vi "Keithley 648X Series Acquire and Enable Relative Values.vi"() -> ()   [LabVIEW 2024]
doc: "This example shows how to configure a measurement and take a reading."
uses:
  <instrlib>/Keithley 648X Series/Keithley 648X Series.lvlib
panel:
  in  "Digital Filter Noise Tolerance":dbl
  in  "Enable Digital Filter":u16(ring) items=["Disable", "Enable", "Advanced"]
  in  "Digital Filter Type":u16(ring) items=["Repeating", "Moving"]
  in  "Digital Filter Count":i32=10
  in  "Median Filter Rank":u16(ring)=1 items=["1"=1, "2"=2, "3"=3, "4"=4, "5"=5]
  in  "Enable Median Filter":bool
  in  "Measurement Time":dbl=6.0
  in  "Trigger Delay":dbl
  in  "Trigger Loop Count":i32=1
  in  "Trigger Source":u16(ring) items=["Immediate", "Tlink"]
  in  "Arm Timer Interval":dbl=0.1
  in  "Arm Loop Count":i32=1
  in  "Arm Source":u16(ring) items=["Immediate", "Timer", "Bus", "Tlink", "Manual", "Negative SOT", "Positive SOT", "Bidirectional SOT"]
  out "Relative Measurements":cluster{dbl[], dbl[]}(graph)
  in  "Serial Configuration":T1={"Baud Rate"=9600, "Parity"=0, "Data Bits"=8, "Stop Bits"=10, "Flow Control"=0} {"Flow Control" items=["None", "XON/XOFF", "RTS/CTS", "XON/XOFF & RTS/CTS", "DTR/DSR", "XON/XOFF & DTR/DSR"]; "Stop Bits" items=["1.0"=10, "1.5"=15, "2.0"=20]; "Data Bits" items=["7"=7, "8"=8]; "Parity" items=["None", "Odd", "Even", "Mark", "Space"]; "Baud Rate" items=["300"=300, "600"=600, "1200"=1200, "2400"=2400, "4800"=4800, "9600"=9600, "19200"=19200]}
  in  "VISA resource name":refnum<visa-resource-name>
  # "(c) 2017 National Instruments.  ALL RIGHTS RESERVED."
  # "Note: The product of Arm Loop Count and Trigger Loop Count cannot exceed the maximum non-infinite value that either control can take."
  # "Configure Data Acquisition"
  # "Configure Data Filtration"
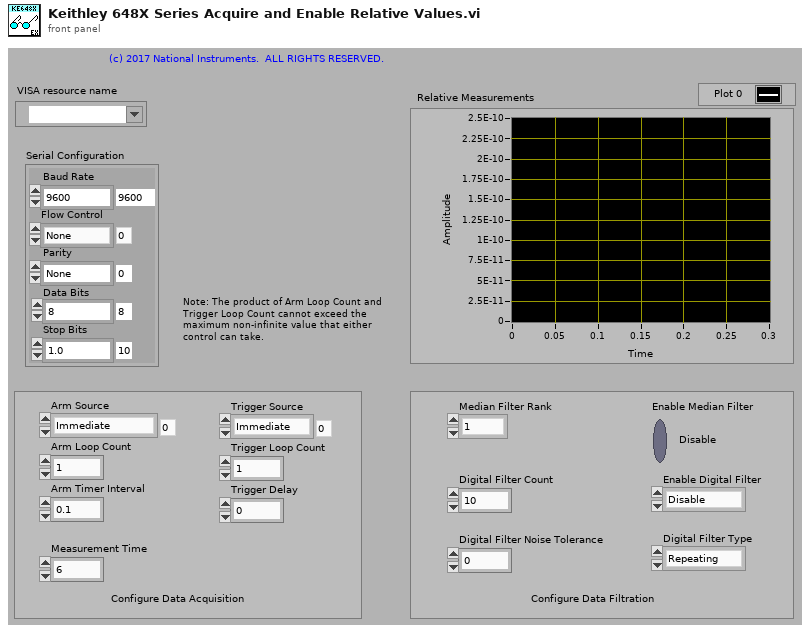
[diagram p1: front panel]
types:
  T1 = cluster{"Baud Rate":u32, "Parity":u16, "Data Bits":u16, "Stop Bits":u16, "Flow Control":u16}
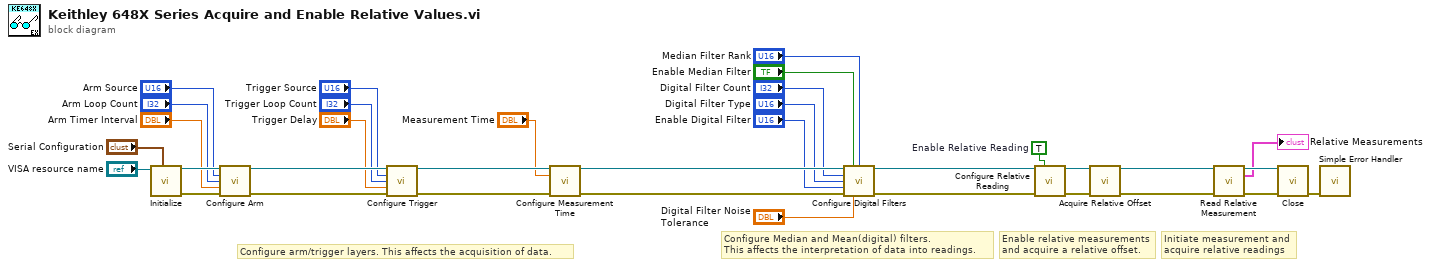
[diagram p0: block diagram]
diagram:
  w20 = TRUE  # Enable Relative Reading
  # "Initiate measurement and\nacquire relative readings"
  # "Enable relative measurements\nand acquire a relative offset."
  # "Configure Median and Mean(digital) filters.\nThis affects the interpretation of data into readings."
  # "Configure arm/trigger layers. This affects the acquisition of data."
  n1 = call <instrlib>:"Initialize.vi"("Serial Configuration"="Serial Configuration", "VISA resource name"="VISA resource name") -> ("error out"=w30:errorcluster, "VISA resource name out"=w29:refnum<visa-resource-name>)  [unwired: 8 in]
  n2 = call <instrlib>:"Configure Arm.vi"("VISA resource name"=w29, "Arm Source (0: Immediate)"="Arm Source", "Arm Loop Count (1)"="Arm Loop Count", "Arm Timer Interval (0.1 s)"="Arm Timer Interval", "error in (no error)"=w30) -> ("VISA resource name out"=w28:refnum<visa-resource-name>, "error out"=w31:errorcluster)  [unwired: 9 in]
  n3 = call <instrlib>:"Configure Trigger.vi"("VISA resource name"=w28, "Trigger Source (0: Immediate)"="Trigger Source", "Trigger Loop Count (1)"="Trigger Loop Count", "Trigger Delay (0 s)"="Trigger Delay", "error in (no error)"=w31) -> ("VISA resource name out"=w13:refnum<visa-resource-name>, "error out"=w12:errorcluster)  [unwired: 9 in]
  n4 = call <instrlib>:"Configure Measurement Time.vi"("VISA resource name"=w13, "Measurement Time (6 PLC)"="Measurement Time", "error in (no error)"=w12) -> ("VISA resource name out"=w10:refnum<visa-resource-name>, "error out"=w9:errorcluster)  [unwired: 11 in]
  n5 = call <instrlib>:"Configure Digital Filters.vi"("VISA resource name"=w10, "Enable Median Filter (F: Disable)"="Enable Median Filter", "Median Filter Rank (1)"="Median Filter Rank", "Digital Filter Count (10)"="Digital Filter Count", "Digital Filter Type (0: Repeating)"="Digital Filter Type", "Enable Digital Filter (0: Disable)"="Enable Digital Filter", "error in (no error)"=w9, "Digital Filter Noise Tolerance (0%)"="Digital Filter Noise Tolerance") -> ("VISA resource name out"=w7:refnum<visa-resource-name>, "error out"=w8:errorcluster)  [unwired: 6 in]
  n6 = call <instrlib>:"Configure Relative Reading.vi"("VISA resource name"=w7, "Enable Relative Reading (F: Disable)"=w20, "error in (no error)"=w8) -> ("VISA resource name out"=w27:refnum<visa-resource-name>, "error out"=w26:errorcluster)  [unwired: 11 in]
  n7 = call <instrlib>:"Acquire Relative Offset.vi"("VISA resource name"=w27, "error in (no error)"=w26) -> ("VISA resource name out"=w24:refnum<visa-resource-name>, "error out"=w25:errorcluster)  [unwired: 12 in]
  n8 = call <instrlib>:"Read Relative Measurement.vi"("VISA resource name"=w24, "error in (no error)"=w25) -> ("VISA resource name out"=w23:refnum<visa-resource-name>, "Relative Measurements"=→"Relative Measurements":cluster{dbl[], dbl[]}, "error out"=w22:errorcluster)  [unwired: 11 in]
  n9 = call <instrlib>:"Close.vi"("error in (no error)"=w22, "VISA resource name"=w23) -> ("error out"=w34:errorcluster)  [unwired: 9 in]
  n10 = call <vilib>:"Simple Error Handler.vi"("error in (no error)"=w34) -> ()  [unwired: 4 in, 5 out]
